vi "Unflatten Linked List.vi"(6 "Flattened Linked List":string, 7 "Parent ID":string, 8 "error in (no error)":errorcluster, 10 "Persistence":refnum<class "IPersist.lvclass">, 11 "Linked List Ref":refnum<data-value>) -> (0 "error out":errorcluster, 3 "Linked List Ref out":refnum<data-value>, 5 "Linked List ID out":string)   [LabVIEW 2020, in "Linked Lists.lvlib" / "Linked List Ref.lvclass"]
uses:
  <vilib>/gpm_packages/@cs/linked-list/Source/Linked List/Linked List Ref/Linked List Ref.lvclass
  <vilib>/gpm_packages/@cs/linked-list/Source/Linked List/ILinkedList/ILinked List.lvclass
  <vilib>/gpm_packages/@cs/persistence/source/IPersist/IPersist.lvclass
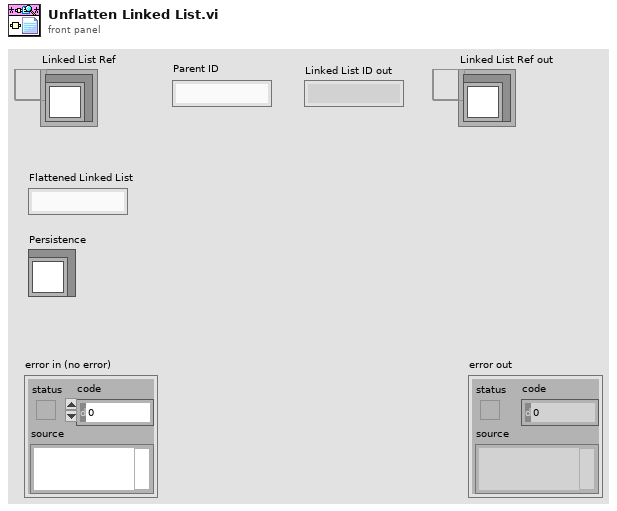
[diagram p1: front panel]
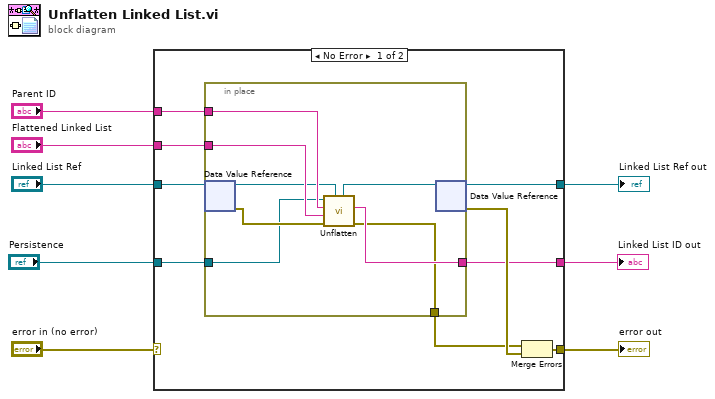
[diagram p0: block diagram]
diagram:
  n1 = case shown="No Error" "error in (no error)" {
    selector: "error in (no error)" -> [_ w27]
    tunnel: "Linked List Ref" -> [w17 w26]
    tunnel: "Flattened Linked List" -> [w16 _]
    tunnel: [w14 w27] -> w5
    tunnel: [w15 w26] -> w4
    tunnel: "Parent ID" -> [w11 _]
    tunnel: [w10 _] -> w2
    tunnel: "Persistence" -> [w9 _]
    frame No Error {
      n2 = in-place {
        in-place-border: w16 -> [w24]
        in-place-border: [w18] -> w12
        in-place-border: w11 -> [w23]
        in-place-border: [w22] -> w10
        in-place-border: w9 -> [w20]
        n3 = in-place-dvr #1(w17) -> (w21:refnum<class "ILinked List.lvclass">, w25:errorcluster)
        n4 = call-dynamic "Unflatten.vi"("ILinked List in"=w21, "error in (no error)"=w25, "Flattened Linked List"=w24, "Linked List ID"=w23, "IPersist in"=w20) -> ("error out"=w18:errorcluster, "Linked List ID out"=w22:string, "ILinked List out"=w19:refnum<class "ILinked List.lvclass">)  [unwired: 2 in, 2 out]
        n5 = in-place-dvr #1(w19) -> (w15:refnum<data-value>, w13:errorcluster)
      }
      n6 = Merge Errors(w12, w13) -> (w14:errorcluster)
    }
    frame Error {
    }
  }
  "error out" <- w5
  "Linked List Ref out" <- w4
  "Linked List ID out" <- w2
